vi "set_General.vi"(0 "Host_Reference":refnum<class "HGF_Reference.lvclass">, 2 "timeout in ms (-1)":i32=-1, 5 "error in (no error)":errorcluster) -> (14 "dup Host_Reference":refnum<class "HGF_Reference.lvclass">, 19 "error out":errorcluster)   [LabVIEW 2009, in "MoAgSy.lvlib" / "MoAgSy_Host.lvclass"]
doc: "<B>public</B> VI changes general settings of referenced Host.\n<B>VI frontpanel has to be shown at vi call.</B>\n\nF.Berck@gsi.de\nGSI Darmstadt 2009"
uses:
  MoAgSy_Host.lvclass
  HGF_BaseClasses/HGF_Reference/HGF_Reference.lvclass
panel:
  in  "General Settings":T1
  in  "Cancel":bool
  in  "Apply":bool
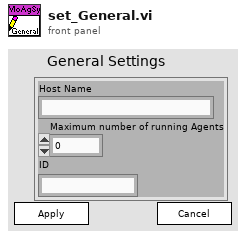
[diagram p1: front panel]
types:
  T1 = cluster{"Host Name":string, "Maximum number of running Agents":i16, "ID":string}
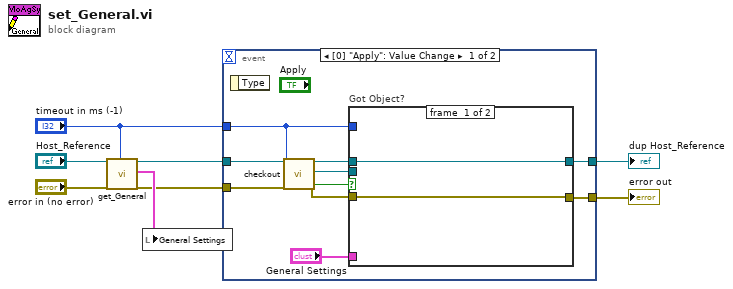
[diagram p0: block diagram]
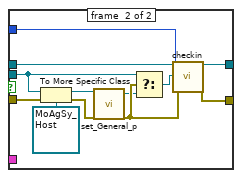
[diagram p2: hidden frame]
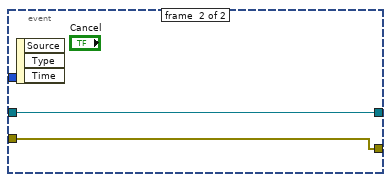
[diagram p3: hidden frame]
diagram:
  n1 = call "get_General.vi"("Host_Reference"="Host_Reference", "timeout in ms (-1)"="timeout in ms (-1)", "error in (no error)"="error in (no error)") -> ("dup Host_Reference"=w5:refnum<class "HGF_Reference.lvclass">, "General"=w4:T1, "error out"=w3:errorcluster)  [unwired: 14 out]
  n2 = local write "General Settings"(w4) -> ()
  n3 = event shown="[0] \"Apply\": Value Change" {
    selector: _ -> [_ _]
    dyn-events: _ -> [_ _]
    timeout: _ -> [_ _]
    tunnel: [w18 w33] -> w7
    tunnel: [w17 w34] -> w8
    tunnel: "timeout in ms (-1)" -> [w13 _]
    tunnel: w5 -> [w12 w34]
    tunnel: w3 -> [w11 w33]
    event #0 {
      n4 = event-data() -> ()  [unwired: 2 out]
      n5 = call "checkout.vi"("HGF_Reference"=w12, "timeout in ms (-1)"=w13, "error in (no error)"=w11) -> ("dup HGF_Reference"=w16:refnum<class "HGF_Reference.lvclass">, "Object"=w14:refnum<class>, "got object?"=w15:bool, "error out"=w10:errorcluster)  [unwired: 13 out]
      n6 = case "Got Object?" shown="True" w15 {
        tunnel: w14 -> [_ w23]
        tunnel: w16 -> [w20 w30]
        tunnel: [w20 w29] -> w17
        tunnel: w13 -> [_ w28]
        tunnel: [w19 w27] -> w18
        tunnel: "General Settings" -> [_ _]
        tunnel: w10 -> [w19 w26]
        frame #0 {
        }
        frame #1 {
          n7 = To More Specific Class(target class=refnum<class "MoAgSy_Host.lvclass"> refnum ("MoAgSy.lvlib:MoAgSy_Host.lvclass"), reference=w23, error in=w26) -> (specific class reference=w25:refnum<class "MoAgSy_Host.lvclass">, error out=w24:errorcluster)
          n8 = call "set_General_p.vi"("MoAgSy_Host"=w25, "error in (no error)"=w24) -> ("dup MoAgSy_Host"=w22:refnum<class "MoAgSy_Host.lvclass">, "error out"=w32:errorcluster)  [unwired: 1 in, 15 out]
          n9 = Select(t=w23, s=w32, f=w22) -> (s? t:f=w21:refnum<class>)
          n10 = call "checkin.vi"("HGF_Reference"=w30, "Object"=w21, "timeout /ms (-1)"=w28, "error in (no error)"=w32) -> ("dup HGF_Reference"=w29:refnum<class "HGF_Reference.lvclass">, "error out"=w27:errorcluster)  [unwired: 14 out]
        }
      }
    }
    event #1 {
      n11 = event-data() -> ()  [unwired: 4 out]
    }
  }
  "dup Host_Reference" <- w8
  "error out" <- w7
